vi "CASE SRTUCTURE with STRING.vi"() -> ()   [LabVIEW 2018]
panel:
  in  "String":string
  out "GREEN":bool
  out "YELLOW":bool
  out "RED":bool
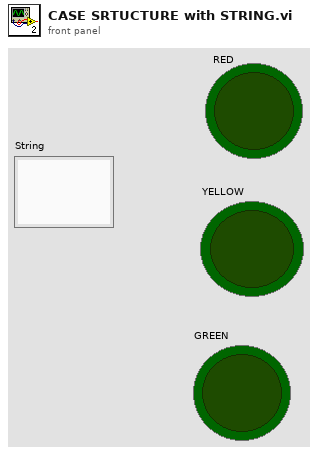
[diagram p1: front panel]
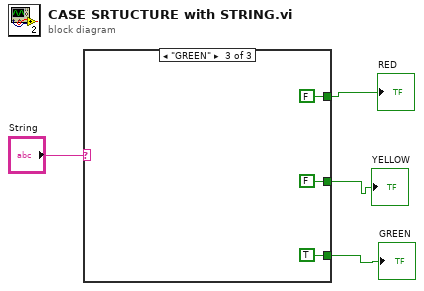
[diagram p0: block diagram]
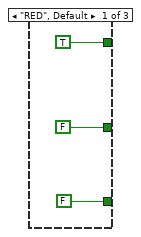
[diagram p2: hidden frame]
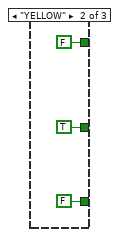
[diagram p3: hidden frame]
diagram:
  n1 = case shown="\"GREEN\"" "String" {
    tunnel: [TRUE FALSE FALSE] -> w3
    tunnel: [FALSE TRUE FALSE] -> w2
    tunnel: [FALSE FALSE TRUE] -> w1
    frame "RED", Default {
    }
    frame "YELLOW" {
    }
    frame "GREEN" {
    }
  }
  "RED" <- w3
  "YELLOW" <- w2
  "GREEN" <- w1
